vi "Compute Target Distances.vi"(10 "Target Info":T4(array[cluster]), 11 "Image in":T3) -> (0 "Distances":T2(array[cluster]), 2 "Target Info":T5(array[cluster]), 3 "Image out":T3)   [LabVIEW 2013]
uses:
  TargetType.ctl
  <vilib>/vision/Image Controls.llb/IMAQ Image.ctl
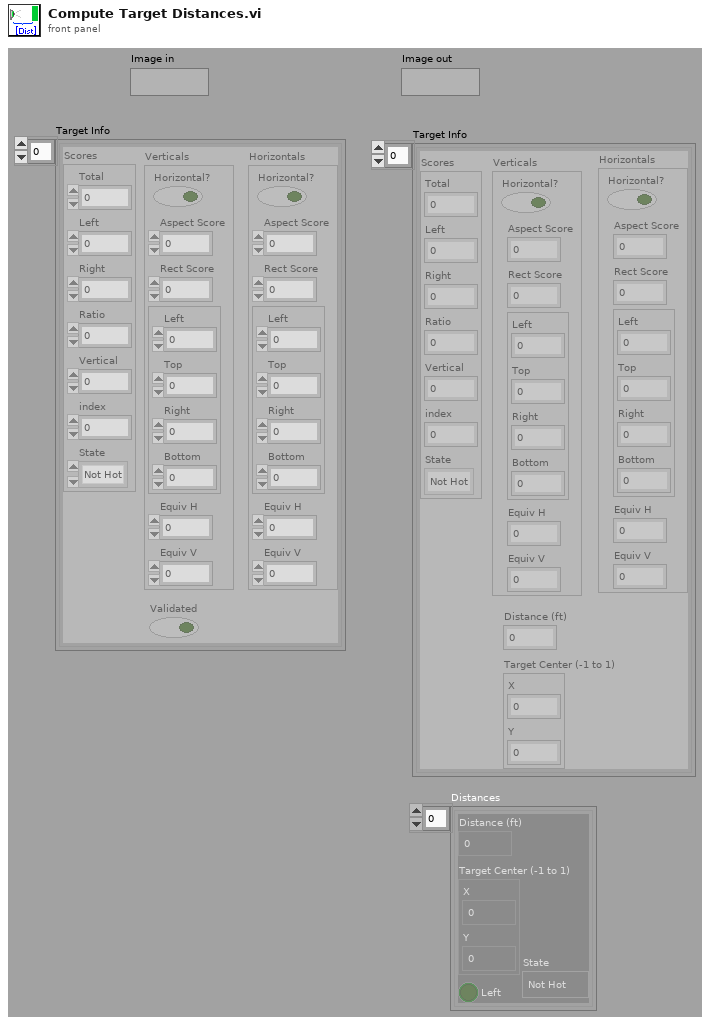
[diagram p1: front panel]
types:
  T1 = typedef "TargetType.ctl" = enum16{"Not Hot", "Hot"}
  T2 = cluster{"Distance (ft)":dbl, "Target Center (-1 to 1)":cluster{"X":dbl, "Y":dbl}, "Left":bool, "State":T1}[]
  T3 = typedef "IMAQ Image.ctl" = refnum<image>
  T4 = cluster{"Scores":cluster{"Total":dbl, "Left":dbl, "Right":dbl, "Ratio":dbl, "Vertical":dbl, "index":i32, "State":T1}, "Verticals":cluster{"Horizontal?":bool, "Aspect Score":dbl, "Rect Score":dbl, cluster{"Left":dbl, "Top":dbl, "Right":dbl, "Bottom":dbl}, "Equiv H":dbl, "Equiv V":dbl}, "Horizontals":cluster{"Horizontal?":bool, "Aspect Score":dbl, "Rect Score":dbl, cluster{"Left":dbl, "Top":dbl, "Right":dbl, "Bottom":dbl}, "Equiv H":dbl, "Equiv V":dbl}, "Validated":bool}[]
  T5 = cluster{"Scores":cluster{"Total":dbl, "Left":dbl, "Right":dbl, "Ratio":dbl, "Vertical":dbl, "index":i32, "State":T1}, "Verticals":cluster{"Horizontal?":bool, "Aspect Score":dbl, "Rect Score":dbl, cluster{"Left":dbl, "Top":dbl, "Right":dbl, "Bottom":dbl}, "Equiv H":dbl, "Equiv V":dbl}, "Horizontals":cluster{"Horizontal?":bool, "Aspect Score":dbl, "Rect Score":dbl, cluster{"Left":dbl, "Top":dbl, "Right":dbl, "Bottom":dbl}, "Equiv H":dbl, "Equiv V":dbl}, "Distance (ft)":dbl, "Target Center (-1 to 1)":cluster{"X":dbl, "Y":dbl}}[]
  T6 = cluster{"Total":dbl, "Left":dbl, "Right":dbl, "Ratio":dbl, "Vertical":dbl, "index":i32, "State":T1}
  T7 = cluster{"Horizontal?":bool, "Aspect Score":dbl, "Rect Score":dbl, cluster{"Left":dbl, "Top":dbl, "Right":dbl, "Bottom":dbl}, "Equiv H":dbl, "Equiv V":dbl}
  T8 = cluster{"Scores":cluster{"Total":dbl, "Left":dbl, "Right":dbl, "Ratio":dbl, "Vertical":dbl, "index":i32, "State":T1}, "Verticals":cluster{"Horizontal?":bool, "Aspect Score":dbl, "Rect Score":dbl, cluster{"Left":dbl, "Top":dbl, "Right":dbl, "Bottom":dbl}, "Equiv H":dbl, "Equiv V":dbl}, "Horizontals":cluster{"Horizontal?":bool, "Aspect Score":dbl, "Rect Score":dbl, cluster{"Left":dbl, "Top":dbl, "Right":dbl, "Bottom":dbl}, "Equiv H":dbl, "Equiv V":dbl}, "Distance (ft)":dbl, "Target Center (-1 to 1)":cluster{"X":dbl, "Y":dbl}}
  T9 = cluster{"Distance (ft)":dbl, "Target Center (-1 to 1)":cluster{"X":dbl, "Y":dbl}, bool, "State":T1}
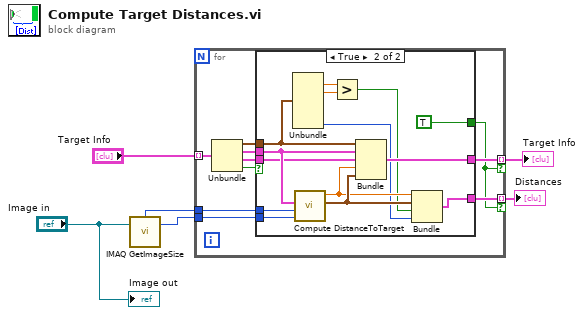
[diagram p0: block diagram]
diagram:
  n1 = call "IMAQ GetImageSize"("Image"="Image in") -> ("Y Resolution"=w5:i32, "X Resolution"=w4:i32)  [unwired: 3 in, 1 out]
  n2 = for {
    tunnel: "Target Info" -> [w16] mode=indexing
    tunnel: w4 -> [w13]
    tunnel: w5 -> [w12]
    tunnel: [w9] -> w6 mode=indexing if=w7
    tunnel: [w8] -> w1 mode=indexing if=w7
    n3 = Unbundle(w16) -> ("Scores"=w11:T6, "Verticals"=w14:T7, "Horizontals"=w10:T7, "Validated"=w15:bool)
    n4 = case shown="True" w15 {
      tunnel: w14 -> [_ w28]
      tunnel: w13 -> [_ w30]
      tunnel: w12 -> [_ w29]
      tunnel: w11 -> [_ w21]
      tunnel: w10 -> [_ w27]
      tunnel: [_ w26] -> w9
      tunnel: [_ TRUE] -> w7
      tunnel: [_ w22] -> w8
      frame False {
      }
      frame True {
        n5 = Unbundle(w21) -> ("Left"=w20:dbl, "Right"=w19:dbl, "State"=w17:T1)  [unwired: 4 out]
        n6 = call "Compute DistanceToTarget.vi"("Y Image Resolution"=w29, "X Image Resolution"=w30, "Vertical Strip"=w28) -> ("Target Center (-1 to 1)"=w24:cluster{"X":dbl, "Y":dbl}, "Distance (ft)"=w23:dbl)  [unwired: 7 in]
        n7 = Greater?(x=w20, y=w19) -> (0:w18:bool)
        n8 = Bundle("Scores"=w21, "Verticals"=w28, "Horizontals"=w27, "Distance (ft)"=w23, "Target Center (-1 to 1)"=w24) -> (w26:T8)  [unwired: 1 in]
        n9 = Bundle("Distance (ft)"=w23, "Target Center (-1 to 1)"=w24, w18, "State"=w17) -> (w22:T9)  [unwired: 1 in]
      }
    }
  }
  "Target Info" <- w6
  "Distances" <- w1
  "Image out" <- "Image in"
